vi "Configure Serial Bus Lister.vi"(8 "error in (no error)":errorcluster, 9 "Time Reference (0: Trigger)":i32(ring) items=["Trigger", "Previous"], 10 "Serial Bus Lister Display (0: Off)":i32(ring) items=["Off", "Serial Bus 1", "Serial Bus 2", "All"], 11 "VISA resource name":refnum<visa-resource-name>) -> (0 "error out":errorcluster, 3 "VISA resource name out":refnum<visa-resource-name>)   [LabVIEW 2023, in "Keysight-DSQx3014T.lvlib"]
doc: "Configures the serial bus lister."
uses:
  Keysight-DSQx3014T.lvlib
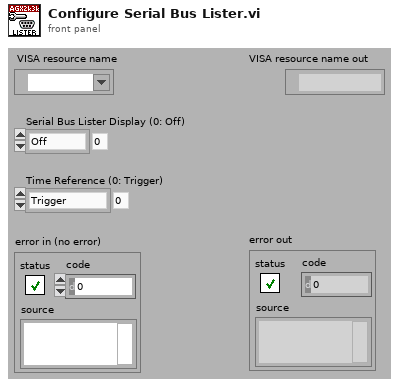
[diagram p1: front panel]
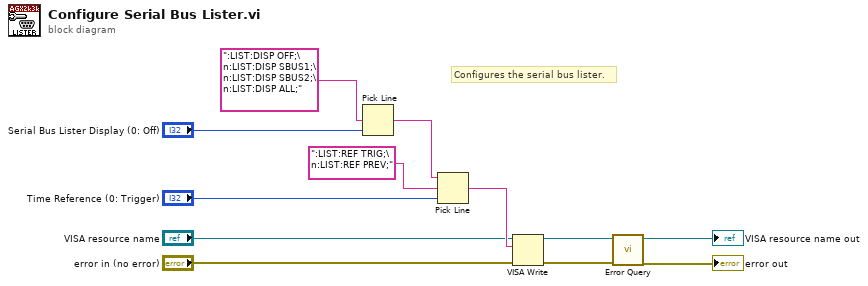
[diagram p0: block diagram]
diagram:
  # "Configures the serial bus lister."
  n1 = Pick Line(multi-line string=":LIST:DISP OFF;\n:LIST:DISP SBUS1;\n:LIST:DISP SBUS2;\n:LIST:DISP ALL;", line index="Serial Bus Lister Display (0: Off)") -> (output string=w8:string)  [unwired: 1 out]
  n2 = Pick Line(string ("")=w8, multi-line string=":LIST:REF TRIG;\n:LIST:REF PREV;", line index="Time Reference (0: Trigger)") -> (output string=w7:string)
  n3 = VISA Write(VISA resource name="VISA resource name", write buffer=w7, error in (no error)="error in (no error)") -> (VISA resource name out=w4:refnum<visa-resource-name>, error out=w3:errorcluster)  [unwired: 1 out]
  n4 = call "Error Query.vi"("error in (no error)"=w3, "VISA resource name"=w4) -> ("error out"=→"error out":errorcluster, "VISA resource name out"=→"VISA resource name out":refnum<visa-resource-name>)  [unwired: 8 out]
